vi "N-Double FFT Mesurament RT Test (OK fino a 8 signals).vi"() -> ()   [LabVIEW 2014]
uses:
  <vilib>/Platform/TimedLoop/XDataNode/timing_clust.ctl
  <vilib>/Platform/TimedLoop/XDataNode/nitl_modes.ctl
  <vilib>/Platform/TimedLoop/XDataNode/wakeup.ctl
  <vilib>/FPGAPlugInAG/sbRIO-9636/niLvFpga_Open_sbRIO-9636.vi
  <vilib>/rvi/interface/common/dynamic/niFpgaDynamicAddResources.vi
  <vilib>/FPGAPlugInAG/Dynamic/niLvFpga_Reset_Dynamic.vi
  <vilib>/Utility/error.llb/Error Cluster From Error Code.vi
  <vilib>/rvi/errors/niLvFpgaAdjustHostInterfaceError.vi
  <vilib>/rvi/interface/common/niFpgaWaitOnOcc.vi
  <vilib>/FPGAPlugInAG/Dynamic/niLvFpga_Run_Dynamic.vi
  <vilib>/FPGAPlugInAG/Dynamic/niLvFpga_Abort_Dynamic.vi
  <vilib>/FPGAPlugInAG/Dynamic/niLvFpga_Close_Dynamic.vi
  <vilib>/rvi/interface/nirviOpenFPGA/nirviOpenFPGA.xnode
  FPGA Bitfiles/LaserDistanceSen_FPGATarget_N-DoubleFFTMesur_iXckxMnFQJ0.lvbitx
  FPGA Target/Test VIs/N-Double FFT Mesurament (N-Parametric ALTERNATIVE) Test.vi
  <vilib>/rvi/interface/nirviMethod/nirviMethod.xnode
  <vilib>/rvi/interface/nirviReadWriteControl/nirviReadWriteControl.xnode
  <vilib>/platform/TimedLoop/XDataNode/XDataNode.xnode
  <vilib>/rvi/interface/nirviCloseFPGA/nirviCloseFPGA.xnode
  <vilib>/FPGAPlugInAG/Dynamic/niLvFpga_ConfigureFifo_Dynamic.vi
  <vilib>/rvi/errors/niLvFpgaMergeErrorWithErrorCode.vi
  <vilib>/FPGAPlugInAG/Dynamic/niLvFpga_StartFifo_Dynamic.vi
  <vilib>/rvi/interface/Simulation/niFpgaSimulationCallBeginRW.vi
  <vilib>/FPGAPlugInAG/Dynamic/niLvFpga_ReadFifo_Dynamic.vi
  NiFpgaLv.dll
  <vilib>/Platform/TimedLoop/XDataNode/XDNodeRunTimeDep.lvlib
panel:
  out "error out":errorcluster
  out "N-FFT":dbl[](graph)
  out "Write memory complete":bool
  in  "#Signals":u32=5
  in  "stop":bool
  in  "Initial Latency points":u32(slide) scale=0.0..1249.0
  out "Elements Remaining FFT":u32
  out "Elements Remaining Signal":u32
  out "N-Signals":dbl[](graph)
  in  "Snapshot":bool
  in  "Windowing":T1(ring)
  in  "first bin":i32=15
  in  "last bin":i32=255
  in  "lower limit 2":u32(slide)=738 scale=625.0..738.0
  in  "lower limit 1":u32(slide)=113 scale=0.0..113.0
  # "WARNING:\nOnce pressed wait untill the end of operation"
  # "OFFLINE parameters"
  # ">= 9 Signals fa timeout"
  # "Max Detection FFT bin range"
  # "TEST"
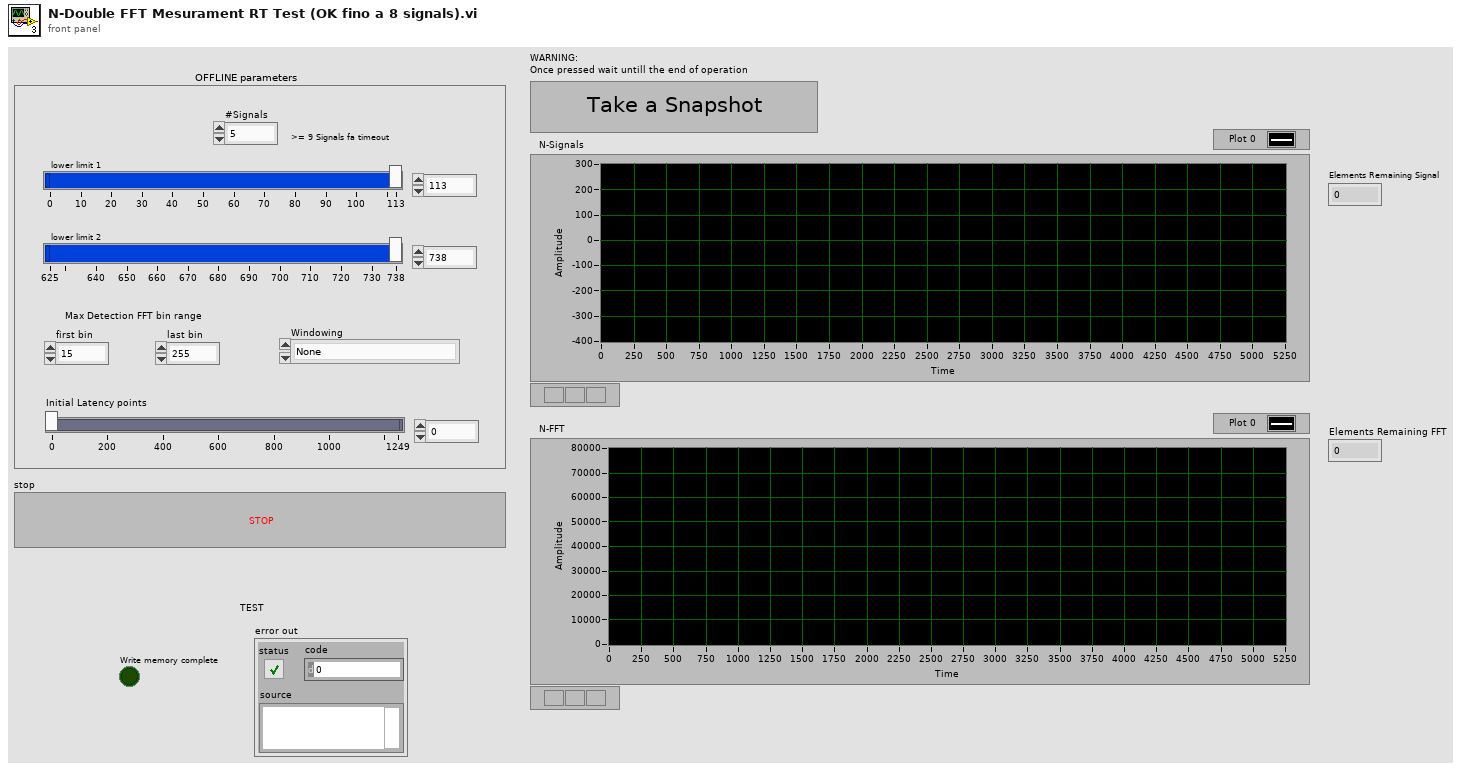
[diagram p1: front panel]
types:
  T1 = enum16{"None", "Hanning", "Hamming", "Blackman", "Blackman-Harris"}
  T2 = typedef "XDNodeRunTimeDep.lvlib/timing_clust.ctl" = cluster{"Expected End [f-1]":u64, "Actual End [f-1]":u64, "Finished Late? [f-1]":bool, "Expected End [i-1]":u64, "Actual End [i-1]":u64, "Finished Late? [i-1]":bool, "Expected Start [i]":u64, "Actual Start [i]":u64, "Expected Start [f]":u64, "Actual Start [f]":u64, "Source Name":string, "Structure Name":string, "Period":i64, "Deadline":i64, "Offset":i64, "Start":i64, "Priority":i32, "Timeout":i32, "Mode":T3, "Wakeup Reason":T4, "Error":errorcluster, "Source Type":string, "Secondary Source Type":string, "Global End Time":u64, "Global Start Time":u64, "Frame Duration":u64, "Iteration Duration":u64, "Assigned CPU":i32, "I/O Scan Engine Mode":u32}
  T3 = typedef "XDNodeRunTimeDep.lvlib/nitl_modes.ctl" = enum32{"No Change", "Process missed periods, maintain original phase", "Discard missed periods, maintain original phase", "Process missed periods, ignore original phase", "Discard missed periods, ignore original phase"}
  T4 = typedef "XDNodeRunTimeDep.lvlib/wakeup.ctl" = enum32{"Normal", "Aborted", "Asynchronous wakeup", "Timing source error", "Timed loop error", "Timeout"}
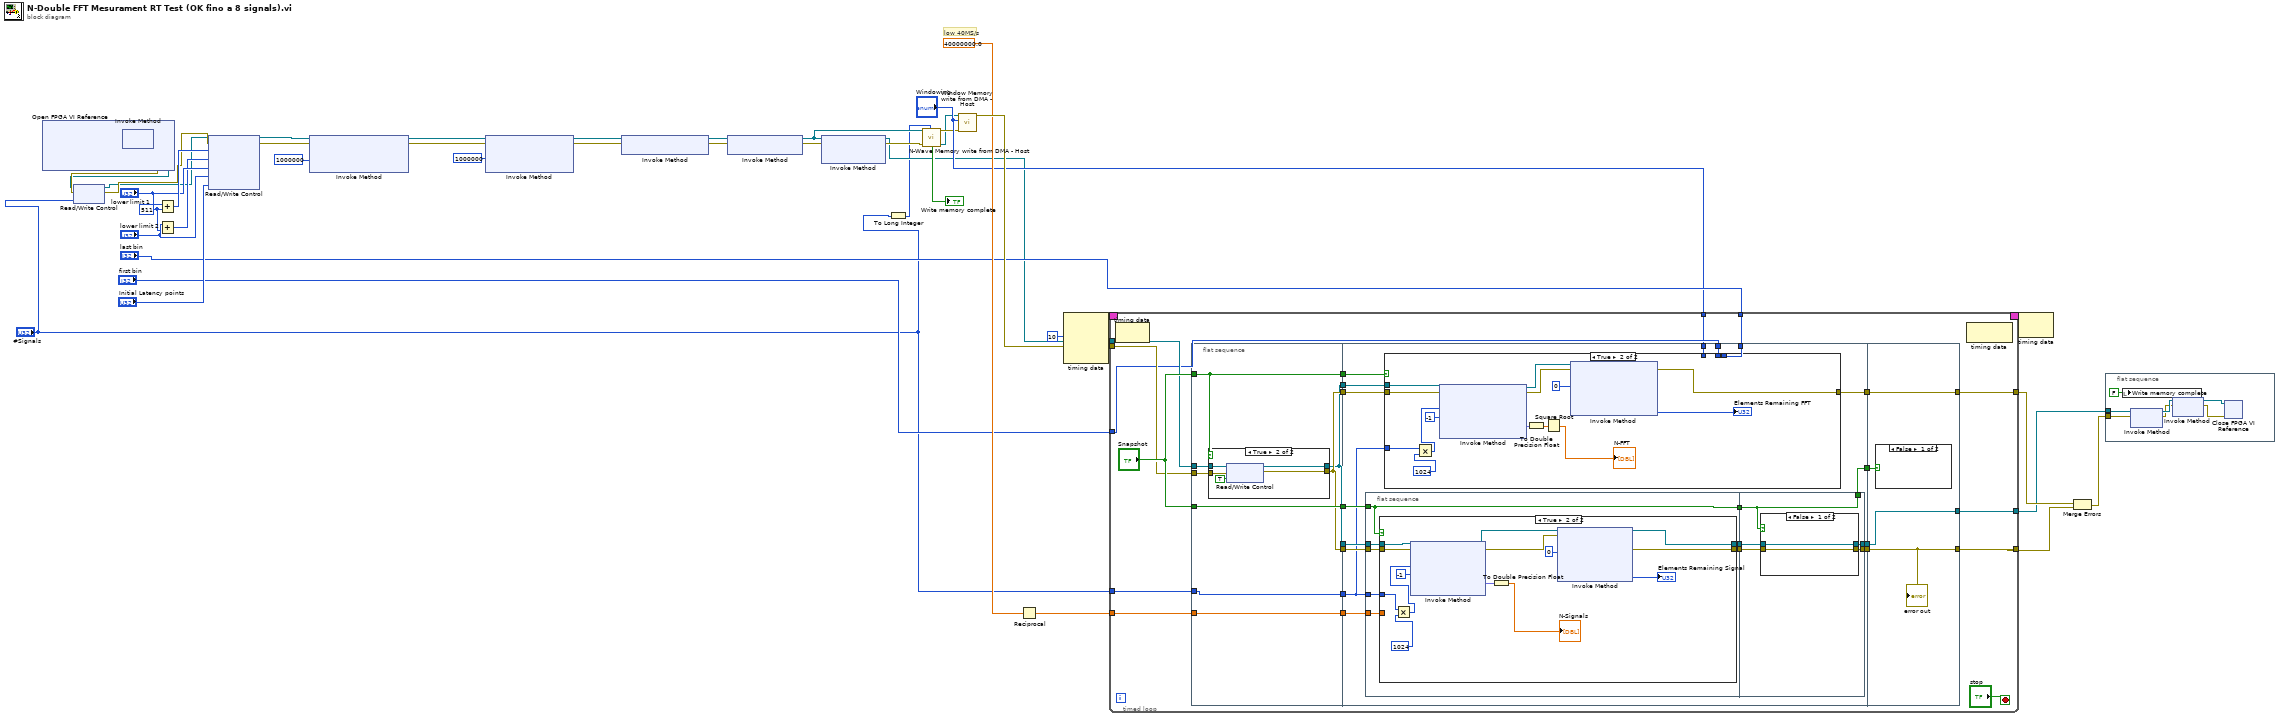
[diagram p0: block diagram]
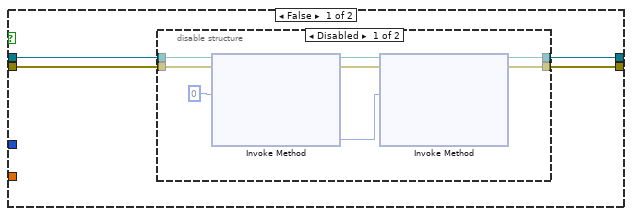
[diagram p3: hidden frame]
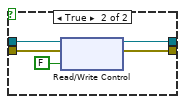
[diagram p5: hidden frame]
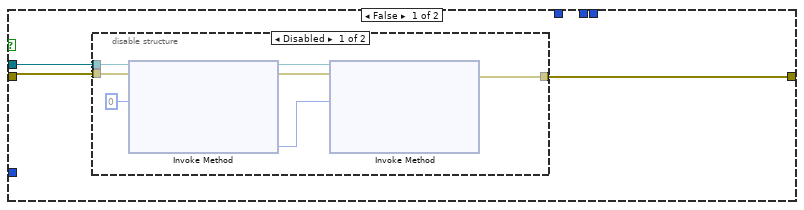
[diagram p6: hidden frame]
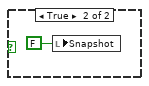
[diagram p8: hidden frame]
diagram:
  w40 = u32 511 ("y")
  # "low 40MS/s"
  n1 = xnode "Open FPGA VI Reference"() -> ("FPGA VI Reference Out"=w7:refnum<k20>, "error out"=w6:errorcluster)  [unwired: 2 in]
  n2 = xnode "Invoke Method"("FPGA VI Reference In"=w7, "error in"=w6) -> ("FPGA VI Reference Out"=w2:refnum<k20>, "error out"=w4:errorcluster)
  n3 = xnode "Read/Write Control"("FPGA VI Reference In"=w2, "error in"=w4, "n"="#Signals") -> ("FPGA VI Reference Out"=w1:refnum<k20>, "error out"=w3:errorcluster)
  n4 = Add(x="lower limit 1", y=w40) -> (x+y=w44:u32)
  n5 = Add(x="lower limit 2", y=w40) -> (x+y=w42:u32)
  n6 = xnode "Read/Write Control"("FPGA VI Reference In"=w1, "error in"=w3, "upper limit 1"=w44, "upper limit 2"=w42, "lower limit 1"="lower limit 1", "lower limit 2"="lower limit 2", "Latency points"="Initial Latency points") -> ("FPGA VI Reference Out"=w38:refnum<k20>, "error out"=w37:errorcluster)
  n7 = xnode "Invoke Method"("FPGA VI Reference In"=w38, "error in"=w37, "Requested Depth"=u32 1000000) -> ("FPGA VI Reference Out"=w21:refnum<k20>, "error out"=w22:errorcluster)  [unwired: 1 out]
  n8 = xnode "Invoke Method"("FPGA VI Reference In"=w21, "error in"=w22, "Requested Depth"=u32 1000000) -> ("FPGA VI Reference Out"=w30:refnum<k20>, "error out"=w31:errorcluster)  [unwired: 1 out]
  n9 = xnode "Invoke Method"("FPGA VI Reference In"=w30, "error in"=w31) -> ("FPGA VI Reference Out"=w19:refnum<k20>, "error out"=w20:errorcluster)
  n10 = xnode "Invoke Method"("FPGA VI Reference In"=w19, "error in"=w20) -> ("FPGA VI Reference Out"=w12:refnum<k20>, "error out"=w29:errorcluster)
  n11 = xnode "Invoke Method"("FPGA VI Reference In"=w12, "error in"=w29) -> ("FPGA VI Reference Out"=w13:refnum<k20>, "error out"=w17:errorcluster)  [unwired: 1 in]
  n12 = To Long Integer(number="#Signals") -> (32bit integer=w11:i32)
  n13 = call "N-Wave Memory write from DMA - Host.vi"("n"=w11, "error in"=w17, "FPGA VI Reference In"=w12) -> ("FPGA VI Reference Out"=w15:refnum<k20>, "error out"=w16:errorcluster, "Write memory complete"=→"Write memory complete":bool)  [unwired: 6 in]
  n14 = call "Window Memory write from DMA - Host.vi"("error in"=w16, "Enum"="Windowing", "FPGA VI Reference In"=w15) -> ("error out"=w39:errorcluster)  [unwired: 5 in, 3 out]
  n15 = Reciprocal(x=40000000.0 ("Sample Rate (S/s)")) -> (1/x=w33:dbl)
  n16 = node-c288(i64 10 ("Period")) -> (w10:T2)  [unwired: 3 in]
  n17 = timed-loop {
    tunnel: w13 -> [w63]
    tunnel: w39 -> [w64]
    tunnel: [w66] -> w28
    tunnel: w33 -> [w68]
    tunnel: [w67] -> w27
    tunnel: "first bin" -> [w52]
    tunnel: "last bin" -> [w51]
    tunnel: [w49] -> w23
    tunnel: "Windowing" -> [w47]
    tunnel: "#Signals" -> [w45]
    timing: w10 -> [_]
    timing-out: [_] -> w9
    stop <- "stop" stop-if-true
    n18 = node-c288() -> ()  [unwired: 1 in, 1 out]
    n19 = flat-sequence {
      tunnel: w63 -> [w74]
      tunnel: w64 -> [w75]
      tunnel: "Snapshot" -> [w72]
      tunnel: "Snapshot" -> [w77]
      tunnel: w68 -> [w78]
      tunnel: [w76] -> w62
      tunnel: [w78] -> w61
      tunnel: [w77] -> w60
      tunnel: [w72] -> w59
      tunnel: [w76] -> w58
      tunnel: [w73] -> w57
      tunnel: [w73] -> w56
      tunnel: [w71] -> w46
      tunnel: w45 -> [w71]
      tunnel: w62 -> [w99]
      tunnel: w61 -> [w98]
      tunnel: w60 -> [w92]
      tunnel: w59 -> [w95]
      tunnel: w58 -> [w94]
      tunnel: w57 -> [w93]
      tunnel: w56 -> [w100]
      tunnel: [w97] -> w55
      tunnel: [w96] -> w54
      tunnel: [w91] -> w53
      tunnel: w52 -> [w90]
      tunnel: w51 -> [w89]
      tunnel: [w88] -> w48
      tunnel: w47 -> [w87]
      tunnel: w46 -> [w86]
      tunnel: [w178] -> w66
      tunnel: [w179] -> w67
      tunnel: w55 -> [w179]
      tunnel: w54 -> [w178]
      tunnel: w53 -> [w177]
      tunnel: [w176] -> w49
      tunnel: w48 -> [w176]
      frame #0 {
        n20 = case shown="True" w72 {
          tunnel: [w79 w85] -> w76
          tunnel: w75 -> [w79 w84]
          tunnel: w74 -> [w80 w83]
          tunnel: [w80 w82] -> w73
          frame False {
          }
          frame True {
            n21 = xnode "Read/Write Control"("FPGA VI Reference In"=w83, "error in"=w84, "snapshot"=TRUE) -> ("FPGA VI Reference Out"=w82:refnum<k20>, "error out"=w85:errorcluster)
          }
        }
      }
      frame #1 {
        n22 = flat-sequence {
          tunnel: w100 -> [w110]
          tunnel: w99 -> [w109]
          tunnel: w98 -> [w108]
          tunnel: w92 -> [w105]
          tunnel: [w107] -> w103
          tunnel: [w106] -> w102
          tunnel: [w105] -> w101
          tunnel: w86 -> [w104]
          tunnel: [w141] -> w96
          tunnel: w103 -> [w143]
          tunnel: w102 -> [w142]
          tunnel: w101 -> [w140]
          tunnel: [w140] -> w91
          tunnel: [w139] -> w88
          frame #0 {
            n23 = case shown="True" w105 {
              tunnel: w110 -> [w114 w138]
              tunnel: w109 -> [w113 w137]
              tunnel: [w112 w136] -> w106
              tunnel: w108 -> [_ _]
              tunnel: [w111 w135] -> w107
              tunnel: w104 -> [_ w134]
              frame False {
                n24 = disable-structure shown="Disabled" {
                  disable-tunnel: w114 -> [w121 w124]
                  disable-tunnel: w113 -> [w119 w123]
                  disable-tunnel: [w118 w123] -> w112
                  disable-tunnel: [w115 w124] -> w111
                  frame Disabled {
                    n25 = xnode "Invoke Method"("FPGA VI Reference In"=w121, "error in"=w119, "Number of Elements"=u32 0) -> ("FPGA VI Reference Out"=w117:refnum<k20>, "error out"=w116:errorcluster, "Elements Remaining"=w120:u32)  [unwired: 1 in, 1 out]
                    n26 = xnode "Invoke Method"("FPGA VI Reference In"=w117, "error in"=w116, "Number of Elements"=w120) -> ("FPGA VI Reference Out"=w115:refnum<k20>, "error out"=w118:errorcluster)  [unwired: 1 in, 2 out]
                  }
                  frame Enabled {
                  }
                }
              }
              frame True {
                n27 = Multiply(x=w134, y=u32 1024 ("Number of Elements")) -> (x*y=w128:u32)
                n28 = xnode "Invoke Method"("FPGA VI Reference In"=w138, "error in"=w137, "Number of Elements"=w128, "Timeout (ms)"=-1) -> ("FPGA VI Reference Out"=w131:refnum<k20>, "error out"=w130:errorcluster, "Data"=w133:fxp<+/-,12,12>[])  [unwired: 1 out]
                n29 = To Double Precision Float(number=w133) -> (double precision float=→"N-Signals":dbl[])
                n30 = xnode "Invoke Method"("FPGA VI Reference In"=w131, "error in"=w130, "Number of Elements"=u32 0) -> ("FPGA VI Reference Out"=w135:refnum<k20>, "error out"=w136:errorcluster, "Elements Remaining"=→"Elements Remaining Signal":u32)  [unwired: 1 in, 1 out]
              }
            }
          }
          frame #1 {
            n31 = case shown="False" w140 {
              tunnel: [w145 w148] -> w141
              tunnel: w143 -> [w144 w149]
              tunnel: w142 -> [w145 w147]
              tunnel: [w144 w146] -> w139
              frame False {
              }
              frame True {
                n32 = xnode "Read/Write Control"("FPGA VI Reference In"=w149, "error in"=w147, "snapshot"=FALSE) -> ("FPGA VI Reference Out"=w146:refnum<k20>, "error out"=w148:errorcluster)
              }
            }
          }
        }
        n33 = case shown="True" w95 {
          tunnel: w93 -> [w153 w174]
          tunnel: w94 -> [w152 w175]
          tunnel: [w151 w173] -> w97
          tunnel: w90 -> [_ _]
          tunnel: w89 -> [_ _]
          tunnel: w87 -> [_ _]
          tunnel: w86 -> [_ w172]
          frame False {
            n34 = disable-structure shown="Disabled" {
              disable-tunnel: w153 -> [w159 _]
              disable-tunnel: w152 -> [w156 w161]
              disable-tunnel: [w155 w161] -> w151
              frame Disabled {
                n35 = xnode "Invoke Method"("FPGA VI Reference In"=w159, "error in"=w156, "Number of Elements"=u32 0) -> ("FPGA VI Reference Out"=w157:refnum<k20>, "error out"=w154:errorcluster, "Elements Remaining"=w158:u32)  [unwired: 1 in, 1 out]
                n36 = xnode "Invoke Method"("FPGA VI Reference In"=w157, "error in"=w154, "Number of Elements"=w158) -> ("error out"=w155:errorcluster)  [unwired: 1 in, 3 out]
              }
              frame Enabled {
              }
            }
          }
          frame True {
            n37 = Multiply(x=w172, y=u32 1024 ("Number of Elements")) -> (x*y=w164:u32)
            n38 = xnode "Invoke Method"("FPGA VI Reference In"=w174, "error in"=w175, "Number of Elements"=w164, "Timeout (ms)"=-1) -> ("FPGA VI Reference Out"=w168:refnum<k20>, "error out"=w169:errorcluster, "Data"=w171:fxp<+,44,44>[])  [unwired: 1 out]
            n39 = To Double Precision Float(number=w171) -> (double precision float=w170:dbl[])
            n40 = Square Root(x=w170) -> (sqrt(x)=→"N-FFT":dbl[])
            n41 = xnode "Invoke Method"("FPGA VI Reference In"=w168, "error in"=w169, "Number of Elements"=u32 0) -> ("error out"=w173:errorcluster, "Elements Remaining"=→"Elements Remaining FFT":u32)  [unwired: 1 in, 2 out]
          }
        }
      }
      frame #2 {
        n42 = case shown="False" w177 {
          frame False {
          }
          frame True {
            n43 = local write "Snapshot"(FALSE ("Snapshot")) -> ()
          }
        }
        "error out" <- w178
      }
    }
    n44 = node-c288() -> ()  [unwired: 1 in, 1 out]
  }
  n45 = node-c288(w9) -> ()  [unwired: 1 out]
  n46 = Merge Errors(w27, w28) -> (w34:errorcluster)
  n47 = flat-sequence {
    tunnel: w34 -> [w187]
    tunnel: w23 -> [w182]
    frame #0 {
      n48 = local write "Write memory complete"(FALSE ("Write memory complete")) -> ()
      n49 = xnode "Invoke Method"("FPGA VI Reference In"=w182, "error in"=w187) -> ("FPGA VI Reference Out"=w184:refnum<k20>, "error out"=w183:errorcluster)
      n50 = xnode "Invoke Method"("FPGA VI Reference In"=w184, "error in"=w183) -> ("FPGA VI Reference Out"=w185:refnum<k20>, "error out"=w186:errorcluster)
      n51 = xnode "Close FPGA VI Reference"("FPGA VI Reference In"=w185, "error in"=w186) -> ()  [unwired: 1 out]
    }
  }
